vi "HFRR ADV v030 new software.vi"() -> ()   [LabVIEW 2025] (continued)
                n317 = Wait (ms)(milliseconds to wait=u32 1500) -> ()  [unwired: 1 out]
              }
              frame #5 {
                n318 = stacked-sequence {
                  frame #0 {
                    n319 = Wait (ms)(milliseconds to wait=u32 1500) -> ()  [unwired: 1 out]
                  }
                  frame #1 {
                    n320 = local read "Set Temp"() -> (w400:dbl)
                    n321 = Number To Fractional String(number=w400, precision (6)=i16 2) -> (F-format string=w403:string)  [unwired: 2 in]
                    n322 = Concatenate Strings("ST;" ("Command"), w403) -> (w402:string)
                    n323 = local write "Due Write"(w402) -> ()
                  }
                  frame #2 {
                    n324 = Wait (ms)(milliseconds to wait=u32 1500) -> ()  [unwired: 1 out]
                  }
                  frame #3 {
                    n325 = local write "Due Write"("HE;1" ("Command")) -> ()
                  }
                  frame #4 {
                    n326 = Wait (ms)(milliseconds to wait=u32 1500) -> ()  [unwired: 1 out]
                  }
                }
              }
            }
          }
          frame False {
            n327 = stacked-sequence {
              frame #0 {
                n328 = Wait (ms)(milliseconds to wait=u32 1500) -> ()  [unwired: 1 out]
              }
              frame #1 {
                n329 = Concatenate Strings("ST;" ("Command"), "0" ("string")) -> (w410:string)
                n330 = local write "Due Write"(w410) -> ()
              }
              frame #2 {
                n331 = Wait (ms)(milliseconds to wait=u32 1500) -> ()  [unwired: 1 out]
              }
              frame #3 {
                n332 = local write "Due Write"("HE;0" ("Command")) -> ()
              }
              frame #4 {
                n333 = Wait (ms)(milliseconds to wait=u32 1500) -> ()  [unwired: 1 out]
              }
            }
          }
        }
      }
      event "Headen Service Button": Value Change {
        n334 = event-data() -> ()  [unwired: 1 in, 6 out]
        n335 = local read "Headen Service Button"() -> (w415:bool)
        n336 = case shown="True" w415 {
          frame False {
            n337 = property on="Password 3" class="Clust (strict)"("Visible"=FALSE) -> ()  [unwired: 2 in, 2 out]
            n338 = property on="Service Password Log" class="Str"("Visible"=FALSE) -> ()  [unwired: 2 in, 2 out]
          }
          frame True {
            n339 = property on="Password 3" class="Clust (strict)"("Visible"=TRUE) -> ()  [unwired: 2 in, 2 out]
            n340 = property on="Service Password Log" class="Str"("Visible"=TRUE) -> ()  [unwired: 2 in, 2 out]
          }
        }
      }
      event "Password 3.Service Password": Value Change {
        n341 = event-data() -> ()  [unwired: 1 in, 6 out]
        n342 = Unbundle By Name("Password 3") -> ("Service Password"=w422:string)
        n343 = call <vilib>:"Trim Whitespace.vi"("string"=w422) -> ("trimmed string"=w420:string)  [unwired: 1 in]
        n344 = Equal?(x=w420, y="Service@123") -> (x = y?=w421:bool)
        n345 = case shown="False" w421 {
          selector: w421 -> [w425 w427]
          frame False {
            n346 = local write "Service Password enable"(w425) -> ()
            n347 = property on="Service Password Log" class="Str"("Visible"=TRUE) -> ()  [unwired: 2 in, 2 out]
          }
          frame True {
            n348 = property on="Service Password Log" class="Str"("Visible"=FALSE) -> ()  [unwired: 2 in, 2 out]
            "Service Password enable" <- w427
          }
        }
      }
      event "Sign In": Value Change {
        w429 = FALSE ("Visible")
        n349 = event-data() -> ()  [unwired: 1 in, 6 out]
        n350 = property on="About" class="Clust (strict)"("Visible"=w429) -> ()  [unwired: 2 in, 2 out]
        n351 = property on="Password 3" class="Clust (strict)"("Visible"=w429) -> ()  [unwired: 2 in, 2 out]
        n352 = property on="Service Password Log" class="Str"("Visible"=FALSE) -> ()  [unwired: 2 in, 2 out]
      }
      event "Info": Value Change {
        n353 = event-data() -> ()  [unwired: 1 in, 6 out]
        n354 = local read "Info"() -> (w431:bool)
        n355 = case shown="False" w431 {
          frame False {
            n356 = property on="About" class="Clust (strict)"("Visible"=FALSE) -> ()  [unwired: 2 in, 2 out]
          }
          frame True {
            n357 = property on="About" class="Clust (strict)"("Visible"=TRUE) -> ()  [unwired: 2 in, 2 out]
          }
        }
      }
      event "Calibration": Value Change {
        n358 = event-data() -> ()  [unwired: 1 in, 6 out]
        n359 = local read "Calibration"() -> (w435:bool)
        n360 = case shown="False" w435 {
          frame False {
            n361 = property on="Calibration 2" class="TabCtl (strict)"("Visible"=FALSE) -> ()  [unwired: 2 in, 2 out]
            n362 = local write "Cal Password"("" ("Cal Password")) -> ()
          }
          frame True {
            n363 = property on="Calibration 2" class="TabCtl (strict)"("Visible"=TRUE) -> ()  [unwired: 2 in, 2 out]
            n364 = local write "Cal Password"("" ("Cal Password")) -> ()
          }
        }
        n365 = property on="Wrong Password" class="Str"("Visible"=FALSE) -> ()  [unwired: 2 in, 2 out]
      }
      event "Cal Password": Value Change {
        n366 = event-data() -> ()  [unwired: 1 in, 6 out]
        n367 = local read "Cal Password"() -> (w443:string)
        n368 = call <vilib>:"Trim Whitespace.vi"("string"=w443) -> ("trimmed string"=w442:string)  [unwired: 1 in]
        n369 = Equal?(x=w442, y="Cal@321") -> (x = y?=w440:bool)
        n370 = case shown="True" w440 {
          frame False {
            n371 = property on="Wrong Password" class="Str"("Visible"=TRUE) -> ()  [unwired: 2 in, 2 out]
          }
          frame True {
            n372 = property on="Wrong Password" class="Str"("Visible"=FALSE) -> ()  [unwired: 2 in, 2 out]
            n373 = local write "Main Tab"(T2."About" ("Main Tab")) -> ()
            n374 = local write "Cal Password"("" ("Cal Password")) -> ()
            n375 = local write "Main Dashboard Buttons"(T1."About" ("Main Dashboard Buttons")) -> ()
            n376 = property on="Calibration 2" class="TabCtl (strict)"("Visible"=FALSE) -> ()  [unwired: 2 in, 2 out]
            n377 = local write "Calibration"(FALSE ("Calibration")) -> ()
          }
        }
      }
      event "Calibration Selection": Value Change {
        n378 = event-data() -> ()  [unwired: 1 in, 6 out]
        n379 = local read "Calibration Selection"() -> (w452:T8)
        n380 = case shown="\"Stroke Calibration\"" w452 {
          tunnel: [T7."Stroke" ("Main Calibration Tab") T7."Friction" ("Main Calibration Tab") T7."Main" ("Main Calibration Tab") T7."Temperature" ("Main Calibration Tab")] -> w451
          frame "Stroke Calibration" {
          }
          frame "Friction Force Calibration" {
          }
          frame Default {
          }
          frame "Temperature Calibration" {
          }
        }
        n381 = local write "Main Calibration Tab"(w451) -> ()
      }
      event "Back Stroke": Value Change {
        n382 = event-data() -> ()  [unwired: 1 in, 6 out]
        n383 = local write "Main Stroke Tab"(T9."Step 1" ("Main Stroke Tab")) -> ()
        n384 = local write "Main Calibration Tab"(T7."Main" ("Main Calibration Tab")) -> ()
        n385 = local write "Back Stroke"(FALSE ("Back Stroke")) -> ()
      }
      event "Step 2 Back": Value Change {
        n386 = event-data() -> ()  [unwired: 1 in, 6 out]
        n387 = local write "Main Stroke Tab"(T9."Step 1" ("Main Stroke Tab")) -> ()
        n388 = local write "Step 2 Back"(FALSE ("Back Stroke")) -> ()
      }
      event "Step 3 Back": Value Change {
        n389 = event-data() -> ()  [unwired: 1 in, 6 out]
        n390 = local write "Main Stroke Tab"(T9."Step 2" ("Main Stroke Tab")) -> ()
        n391 = local write "Step 3 Back"(FALSE ("Back Stroke")) -> ()
      }
      event "Step 4 Back": Value Change {
        n392 = event-data() -> ()  [unwired: 1 in, 6 out]
        n393 = local write "Main Stroke Tab"(T9."Step 3" ("Main Stroke Tab")) -> ()
        n394 = local write "Step 4 Back"(FALSE ("Back Stroke")) -> ()
      }
      event "Step 5 Back": Value Change {
        n395 = event-data() -> ()  [unwired: 1 in, 6 out]
        n396 = local write "Main Stroke Tab"(T9."Step 4" ("Main Stroke Tab")) -> ()
        n397 = local write "Step 5 Back"(FALSE ("Back Stroke")) -> ()
      }
      event "Step 6 Back": Value Change {
        n398 = event-data() -> ()  [unwired: 1 in, 6 out]
        n399 = local write "Main Stroke Tab"(T9."Step 5" ("Main Stroke Tab")) -> ()
        n400 = local write "Step 6 Back"(FALSE ("Back Stroke")) -> ()
      }
      event "Back Stroke step 7": Value Change {
        n401 = event-data() -> ()  [unwired: 1 in, 6 out]
        n402 = local write "Main Stroke Tab"(T9."Step 6" ("Main Stroke Tab")) -> ()
        n403 = local write "Back Stroke step 7"(FALSE ("Back Stroke")) -> ()
      }
      event "Back Stroke step 8": Value Change {
        n404 = event-data() -> ()  [unwired: 1 in, 6 out]
        n405 = local write "Main Stroke Tab"(T9."Step 7" ("Main Stroke Tab")) -> ()
        n406 = local write "Back Stroke step 8"(FALSE ("Back Stroke")) -> ()
      }
      event "Back Stroke 8": Value Change {
        n407 = event-data() -> ()  [unwired: 1 in, 6 out]
        n408 = local write "MOVE CARRIAGE TO"(0.2 ("MOVE CARRIAGE TO")) -> ()
        n409 = local write "Main Stroke Tab"(T9."Step 1" ("Main Stroke Tab")) -> ()
        n410 = local write "Back Stroke 8"(FALSE ("Back Stroke 8")) -> ()
      }
      event "Continue Stroke": Value Change {
        n411 = event-data() -> ()  [unwired: 1 in, 6 out]
        n412 = local write "Main Stroke Tab"(T9."Step 2" ("Main Stroke Tab")) -> ()
        n413 = local write "Continue Stroke"(FALSE ("Continue Stroke")) -> ()
      }
      event "Continue Stroke step 2": Value Change {
        n414 = event-data() -> ()  [unwired: 1 in, 6 out]
        n415 = local write "Main Stroke Tab"(T9."Step 3" ("Main Stroke Tab")) -> ()
        n416 = local write "Continue Stroke step 2"(FALSE ("Continue Stroke")) -> ()
      }
      event "Continue Stroke step 3": Value Change {
        n417 = event-data() -> ()  [unwired: 1 in, 6 out]
        n418 = local write "Main Stroke Tab"(T9."Step 4" ("Main Stroke Tab")) -> ()
        n419 = local write "Continue Stroke step 3"(FALSE ("Continue Stroke")) -> ()
      }
      event "Continue Stroke step 4": Value Change {
        n420 = event-data() -> ()  [unwired: 1 in, 6 out]
        n421 = local write "Main Stroke Tab"(T9."Step 5" ("Main Stroke Tab")) -> ()
        n422 = local write "Continue Stroke step 4"(FALSE ("Continue Stroke")) -> ()
      }
      event "Continue Stroke step 5": Value Change {
        n423 = event-data() -> ()  [unwired: 1 in, 6 out]
        n424 = local write "Main Stroke Tab"(T9."Step 6" ("Main Stroke Tab")) -> ()
        n425 = local write "Continue Stroke step 5"(FALSE ("Continue Stroke")) -> ()
      }
      event "Continue Stroke step 6": Value Change {
        n426 = event-data() -> ()  [unwired: 1 in, 6 out]
        n427 = local write "Main Stroke Tab"(T9."Step 7" ("Main Stroke Tab")) -> ()
        n428 = local write "Continue Stroke step 6"(FALSE ("Continue Stroke")) -> ()
      }
      event "Continue Stroke step 7": Value Change {
        w491 = FALSE ("0.2mm")
        n429 = event-data() -> ()  [unwired: 1 in, 6 out]
        n430 = local write "0.4 mm"(w491) -> ()
        n431 = local write "0.6 mm"(w491) -> ()
        n432 = local write "1.0 mm"(w491) -> ()
        n433 = local write "1.2 mm"(w491) -> ()
        n434 = local write "0.2 2"(w491) -> ()
        n435 = local write "0.4 2"(w491) -> ()
        n436 = local write "0.6 2"(w491) -> ()
        n437 = local write "0.8 2"(w491) -> ()
        n438 = local write "1.0 2"(w491) -> ()
        n439 = local write "1.2"(w491) -> ()
        n440 = local write "0.2mm"(w491) -> ()
        n441 = local write "0.8mm"(w491) -> ()
        n442 = local write "Main Stroke Tab"(T9."Step 8" ("Main Stroke Tab")) -> ()
        n443 = local write "Continue Stroke step 7"(FALSE ("Continue Stroke")) -> ()
        n444 = local write "Stroke Test Complete"(T10."Test Progress" ("Stroke Test Complete")) -> ()
        "Position Measurment Temp" <- 0.0 ("Position Measurment Temp")
        "Calibration Tare" <- TRUE ("Calibration Tare")
        "MOVE CARRIAGE TO" <- 0.2 ("MOVE CARRIAGE TO")
      }
      event "Continue Stroke step 8": Value Change {
        n445 = event-data() -> ()  [unwired: 1 in, 6 out]
        n446 = local read "LVDT STROKE  Calibration"() -> (w496:dbl)
        n447 = local read "Position Measurment Temp"() -> (w497:dbl)
        n448 = case shown="7" w497 {
          selector: w497 -> [w502 w507 w512 w517 w522 w526 w529 w530]
          tunnel: w496 -> [w498 w503 w508 w513 w518 w523 _ _]
          frame 0, Default {
            w500 = TRUE ("0.2mm")
            n449 = Increment(x=w502) -> (x+1=w501:i32)
            n450 = local write "Position Measurment Temp"(w501) -> ()
            n451 = local write "0.2mm"(w500) -> ()
            n452 = local write "0.2 2"(w500) -> ()
            n453 = local write "MOVE CARRIAGE TO"(0.4 ("MOVE CARRIAGE TO")) -> ()
            "Calibration 0.2" <- w498
          }
          frame 1 {
            w505 = TRUE ("0.4 mm")
            n454 = Increment(x=w507) -> (x+1=w506:i32)
            n455 = local write "Calibration 0.4"(w503) -> ()
            n456 = local write "Position Measurment Temp"(w506) -> ()
            n457 = local write "0.4 mm"(w505) -> ()
            n458 = local write "MOVE CARRIAGE TO"(0.6 ("MOVE CARRIAGE TO")) -> ()
            n459 = local write "0.4 2"(w505) -> ()
          }
          frame 2 {
            w510 = TRUE ("0.6 mm")
            n460 = Increment(x=w512) -> (x+1=w511:i32)
            n461 = local write "Calibration 0.6"(w508) -> ()
            n462 = local write "Position Measurment Temp"(w511) -> ()
            n463 = local write "0.6 2"(w510) -> ()
            n464 = local write "0.6 mm"(w510) -> ()
            n465 = local write "MOVE CARRIAGE TO"(0.8 ("MOVE CARRIAGE TO")) -> ()
          }
          frame 3 {
            w514 = TRUE ("0.6 mm")
            n466 = Increment(x=w517) -> (x+1=w516:i32)
            n467 = local write "Position Measurment Temp"(w516) -> ()
            n468 = local write "MOVE CARRIAGE TO"(1.0 ("MOVE CARRIAGE TO")) -> ()
            n469 = local write "0.8mm"(w514) -> ()
            n470 = local write "0.8 2"(w514) -> ()
            "Calibration 0.8" <- w513
          }
          frame 4 {
            w519 = TRUE ("0.6 mm")
            n471 = Increment(x=w522) -> (x+1=w521:i32)
            n472 = local write "Position Measurment Temp"(w521) -> ()
            n473 = local write "MOVE CARRIAGE TO"(1.2 ("MOVE CARRIAGE TO")) -> ()
            n474 = local write "1.0 mm"(w519) -> ()
            n475 = local write "1.0 2"(w519) -> ()
            "Calibration 1.0" <- w518
          }
          frame 5 {
            w524 = TRUE ("0.6 mm")
            n476 = Increment(x=w526) -> (x+1=w525:i32)
            n477 = local write "Position Measurment Temp"(w525) -> ()
            n478 = local write "1.2 mm"(w524) -> ()
            n479 = local write "1.2"(w524) -> ()
            "Calibration 1.2" <- w523
          }
          frame 6 {
            n480 = Increment(x=w529) -> (x+1=w528:i32)
            n481 = local write "Position Measurment Temp"(w528) -> ()
            n482 = local write "Stroke Test Complete"(T10."Stroke Points Completed" ("Stroke Test Complete")) -> ()
          }
          frame 7 {
            n483 = stacked-sequence {
              tunnel: w530 -> [w531 _ _]
              frame #0 {
                n484 = Increment(x=w531) -> (x+1=w532:i32)
                n485 = local write "Main Stroke Tab"(T9."Step 9" ("Main Stroke Tab")) -> ()
                n486 = local write "Position Measurment Temp"(w532) -> ()
                n487 = Insert Into Array(array=dbl[] [], new element #1=0.2 ("new element/subarray"), new element #2=0.4 ("new element/subarray"), new element #3=0.6 ("new element/subarray"), new element #4=0.8 ("new element/subarray"), new element #5=1.0 ("new element/subarray"), new element #6=1.2 ("new element/subarray")) -> (→"1D stroke":dbl[])  [unwired: 1 in]
                n488 = local read "Calibration 0.2"() -> (w539:dbl)
                n489 = local read "Calibration 0.4"() -> (w538:dbl)
                n490 = local read "Calibration 0.6"() -> (w537:dbl)
                n491 = local read "Calibration 0.8"() -> (w536:dbl)
                n492 = local read "Calibration 1.0"() -> (w535:dbl)
                n493 = local read "Calibration 1.2"() -> (w534:dbl)
                n494 = Insert Into Array(array=dbl[] [], new element #1=w539, new element #2=w538, new element #3=w537, new element #4=w536, new element #5=w535, new element #6=w534) -> (→"Calibrated Voltage Value":dbl[])  [unwired: 1 in]
              }
              frame #1 {
                n495 = local read "calibration values"() -> (w562:dbl[])
                n496 = local read "Calibrated Voltage Value"() -> (w564:dbl[])
                n497 = Index Array(array=w562, index #1=1 ("index"), index #2=3 ("index"), index #3=5 ("index"), index #4=7 ("index"), index #5=9 ("index"), index #6=11 ("index")) -> (element #1=w555:dbl, element #2=w554:dbl, element #3=w553:dbl, element #4=w552:dbl, element #5=w551:dbl, element #6=w550:dbl)
                n498 = local read "1D stroke"() -> (w565:dbl[])
                n499 = for {
                  tunnel: [w574] -> w563 mode=indexing
                  tunnel: w565 -> [w573] mode=indexing
                  tunnel: w564 -> [w572] mode=indexing
                  tunnel: w555 -> [w571]
                  tunnel: w554 -> [w570]
                  tunnel: w553 -> [w569]
                  tunnel: w552 -> [w568]
                  tunnel: w551 -> [w567]
                  tunnel: w550 -> [w566]
                  n500 = formula code="if (stroke == 0.2)\n{\n    if ((voltage >= REF_02 - 0.2) && (voltage <= REF_02 + 0.2))\n        status = 1;\n    else\n        status = 0;\n}\nelse if (stroke == 0.4)\n{\n    if ((voltage >= REF_04 - 0.2) && (voltage <= REF_04 + 0.2))\n        status = 1;\n    else\n        status = 0;\n}\nelse if (stroke == 0.6)\n{\n    if ((voltage >= REF_06 - 0.2) && (voltage <= REF_06 + 0.2))\n        status = 1;\n    else\n        status = 0;\n}\nelse if (stroke == 0.8)\n{\n    if ((voltage >= REF_08 - 0.2) && (voltage <= REF_08 + 0.2))\n        status = 1;\n    else\n        status = 0;\n}\nelse if (stroke == 1.0)\n{\n    if ((voltage >= REF_10 - 0.2) && (voltage <= REF_10 + 0.2))\n        status = 1;\n    else\n        status = 0;\n}\nelse if (stroke == 1.2)\n{\n    if ((voltage >= REF_12 - 0.2) && (voltage <= REF_12 + 0.2))\n        status = 1;\n    else\n        status = 0;\n}\nelse\n{\n    status = 0;\n}"("stroke"=w573, "voltage"=w572, "REF_02"=w571, "REF_04"=w570, "REF_06"=w569, "REF_08"=w568, "REF_10"=w567, "REF_12"=w566) -> ("status"=w574:dbl)
                }
                "Status" <- w563
              }
              frame #2 {
                w581 = 1.0
                n501 = local read "Status"() -> (w588:dbl[])
                n502 = Index Array(array=w588) -> (element #1=w587:dbl, element #2=w586:dbl, element #3=w585:dbl, element #4=w584:dbl, element #5=w583:dbl, element #6=w582:dbl)  [unwired: 6 in]
                n503 = Equal?(x=w586, y=w581) -> (x = y?=w579:bool)
                n504 = Equal?(x=w585, y=w581) -> (x = y?=w578:bool)
                n505 = Equal?(x=w584, y=w581) -> (x = y?=w577:bool)
                n506 = Equal?(x=w583, y=w581) -> (x = y?=w576:bool)
                n507 = Equal?(x=w582, y=w581) -> (x = y?=w575:bool)
                n508 = Equal?(x=w587, y=w581) -> (x = y?=w580:bool)
                n509 = case shown="True" w580 {
                  selector: w580 -> [w599 w600]
                  frame True {
                    n510 = local write "Point 1 - 0.2 mm"(w599) -> ()
                    n511 = property on="Point 1 - 0.2 mm" class="Bool"("Caption.Visible"=w599) -> ()  [unwired: 2 in, 2 out]
                  }
                  frame False {
                    n512 = local write "Point 1 - 0.2 mm"(w600) -> ()
                    n513 = property on="Point 1 - 0.2 mm" class="Bool"("Caption.Visible"=w600) -> ()  [unwired: 2 in, 2 out]
                  }
                }
                n514 = case shown="True" w579 {
                  selector: w579 -> [w597 w598]
                  frame True {
                    n515 = local write "Point 2 - 0.4 mm"(w597) -> ()
                    n516 = property on="Point 2 - 0.4 mm" class="Bool"("Caption.Visible"=w597) -> ()  [unwired: 2 in, 2 out]
                  }
                  frame False {
                    n517 = local write "Point 2 - 0.4 mm"(w598) -> ()
                    n518 = property on="Point 2 - 0.4 mm" class="Bool"("Caption.Visible"=w598) -> ()  [unwired: 2 in, 2 out]
                  }
                }
                n519 = case shown="True" w576 {
                  selector: w576 -> [w591 w592]
                  frame True {
                    n520 = local write "Point 5 - 1.0 mm"(w591) -> ()
                    n521 = property on="Point 5 - 1.0 mm" class="Bool"("Caption.Visible"=w591) -> ()  [unwired: 2 in, 2 out]
                  }
                  frame False {
                    n522 = local write "Point 5 - 1.0 mm"(w592) -> ()
                    n523 = property on="Point 5 - 1.0 mm" class="Bool"("Caption.Visible"=w592) -> ()  [unwired: 2 in, 2 out]
                  }
                }
                n524 = case shown="True" w578 {
                  selector: w578 -> [w595 w596]
                  frame True {
                    n525 = local write "Point 3 - 0.6 mm"(w595) -> ()
                    n526 = property on="Point 3 - 0.6 mm" class="Bool"("Caption.Visible"=w595) -> ()  [unwired: 2 in, 2 out]
                  }
                  frame False {
                    n527 = local write "Point 3 - 0.6 mm"(w596) -> ()
                    n528 = property on="Point 3 - 0.6 mm" class="Bool"("Caption.Visible"=w596) -> ()  [unwired: 2 in, 2 out]
                  }
                }
                n529 = case shown="True" w577 {
                  selector: w577 -> [w593 w594]
                  frame True {
                    n530 = local write "Point 4 - 0.8 mm"(w593) -> ()
                    n531 = property on="Point 4 - 0.8 mm" class="Bool"("Caption.Visible"=w593) -> ()  [unwired: 2 in, 2 out]
                  }
                  frame False {
                    n532 = local write "Point 4 - 0.8 mm"(w594) -> ()
                    n533 = property on="Point 4 - 0.8 mm" class="Bool"("Caption.Visible"=w594) -> ()  [unwired: 2 in, 2 out]
                  }
                }
                n534 = case shown="True" w575 {
                  selector: w575 -> [w589 w590]
                  frame True {
                    n535 = local write "Point 6 - 1.2 mm"(w589) -> ()
                    n536 = property on="Point 6 - 1.2 mm" class="Bool"("Caption.Visible"=w589) -> ()  [unwired: 2 in, 2 out]
                  }
                  frame False {
                    n537 = local write "Point 6 - 1.2 mm"(w590) -> ()
                    n538 = property on="Point 6 - 1.2 mm" class="Bool"("Caption.Visible"=w590) -> ()  [unwired: 2 in, 2 out]
                  }
                }
              }
            }
          }
        }
      }
      event "TEMPERATURE STEP Back 1", "TEMPERATURE STEP Back air Temp": Value Change {
        n539 = event-data() -> ()  [unwired: 1 in, 6 out]
        n540 = stacked-sequence {
          frame #0 {
            n541 = local write "Main Calibration Tab"(T7."Main" ("Main Calibration Tab")) -> ()
          }
          frame #1 {
            n542 = Wait (ms)(milliseconds to wait=u32 1000) -> ()  [unwired: 1 out]
          }
          frame #2 {
            n543 = local write "Due Write"("CAL;END" ("Command")) -> ()
          }
          frame #3 {
            n544 = Wait (ms)(milliseconds to wait=u32 2000) -> ()  [unwired: 1 out]
          }
          frame #4 {
            n545 = local write "Due Write"("CAL;END" ("Command")) -> ()
          }
        }
      }
      event "Temperature Continue Step 1": Value Change {
        n546 = event-data() -> ()  [unwired: 1 in, 6 out]
        n547 = stacked-sequence {
          frame #0 {
            n548 = Wait (ms)(milliseconds to wait=u32 1500) -> ()  [unwired: 1 out]
          }
          frame #1 {
            n549 = local write "Due Write"("CAL;START" ("Command")) -> ()
          }
          frame #2 {
            n550 = Wait (ms)(milliseconds to wait=u32 1500) -> ()  [unwired: 1 out]
          }
          frame #3 {
            n551 = local write "Due Write"("CAL;START" ("Command")) -> ()
          }
          frame #4 {
            n552 = Wait (ms)(milliseconds to wait=u32 2000) -> ()  [unwired: 1 out]
          }
          frame #5 {
          }
          frame #6 {
            n553 = Wait (ms)(milliseconds to wait=u32 2000) -> ()  [unwired: 1 out]
          }
          frame #7 {
            # "CAL;A1;<true_T>"
            n554 = local write "Due Write"("CAL;A1;0" ("Command")) -> ()
          }
          frame #8 {
            n555 = local write "Tab Control 4"(T12."Step 2" ("Tab Control 4")) -> ()
          }
        }
      }
      event "Temperature Continue Step air Step 1": Value Change {
        n556 = event-data() -> ()  [unwired: 1 in, 6 out]
        n557 = stacked-sequence {
          frame #0 {
            n558 = Wait (ms)(milliseconds to wait=u32 1500) -> ()  [unwired: 1 out]
          }
          frame #1 {
            n559 = local write "Due Write"("CAL;START" ("Command")) -> ()
          }
          frame #2 {
            n560 = Wait (ms)(milliseconds to wait=u32 1500) -> ()  [unwired: 1 out]
          }
          frame #3 {
            n561 = local write "Due Write"("CAL;START" ("Command")) -> ()
          }
          frame #4 {
            n562 = Wait (ms)(milliseconds to wait=u32 2000) -> ()  [unwired: 1 out]
          }
          frame #5 {
          }
          frame #6 {
            n563 = Wait (ms)(milliseconds to wait=u32 2000) -> ()  [unwired: 1 out]
          }
          frame #7 {
            # "CAL;A1;<true_T>"
            n564 = local write "Due Write"("CAL;A1;0" ("Command")) -> ()
          }
          frame #8 {
            n565 = local write "Tab Control 4"(T12."Air Step 2" ("Tab Control 4")) -> ()
          }
        }
      }
      event "Temperature Selection": Value Change {
        n566 = event-data() -> ()  [unwired: 1 in, 6 out]
        n567 = local read "Temperature Selection"() -> (w622:T13)
        n568 = case shown="\"Default\", Default" w622 {
          frame "Air Temperature" {
            n569 = local write "Tab Control 4"(T12."Air Step 1" ("Tab Control 4")) -> ()
          }
          frame "Sample Temperature" {
            n570 = local write "Tab Control 4"(T12."Step 1" ("Tab Control 4")) -> ()
          }
          frame "Default", Default {
          }
        }
      }
      event "Temperature Continue Step 2": Value Change {
        n571 = event-data() -> ()  [unwired: 1 in, 6 out]
        n572 = stacked-sequence {
          frame #0 {
            n573 = stacked-sequence {
              frame #0 {
                n574 = Wait (ms)(milliseconds to wait=u32 1500) -> ()  [unwired: 1 out]
              }
              frame #1 {
                # "CAL;A1;<true_T>"
                n575 = local write "Due Write"("CAL;A1;0" ("Command")) -> ()
              }
              frame #2 {
                n576 = Wait (ms)(milliseconds to wait=u32 1500) -> ()  [unwired: 1 out]
              }
              frame #3 {
                # "CAL;A1;<true_T>"
                n577 = local write "Due Write"("CAL;A1;0" ("Command")) -> ()
              }
              frame #4 {
              }
            }
          }
          frame #1 {
            n578 = local write "Tab Control 4"(T12."Step 3" ("Tab Control 4")) -> ()
          }
        }
      }
      event "Temperature Continue Step 5": Value Change {
        n579 = event-data() -> ()  [unwired: 1 in, 6 out]
        n580 = stacked-sequence {
          frame #0 {
            n581 = stacked-sequence {
              frame #0 {
                n582 = Wait (ms)(milliseconds to wait=u32 1500) -> ()  [unwired: 1 out]
              }
              frame #1 {
                # "CAL;A1;<true_T>"
                n583 = local write "Due Write"("CAL;A1;0" ("Command")) -> ()
              }
              frame #2 {
                n584 = Wait (ms)(milliseconds to wait=u32 1500) -> ()  [unwired: 1 out]
              }
              frame #3 {
                # "CAL;A1;<true_T>"
                n585 = local write "Due Write"("CAL;A1;0" ("Command")) -> ()
              }
              frame #4 {
              }
            }
          }
          frame #1 {
            n586 = local write "Tab Control 4"(T12."Air Step 3" ("Tab Control 4")) -> ()
          }
        }
      }
      event "Temperature Continue Step 3": Value Change {
        n587 = event-data() -> ()  [unwired: 1 in, 6 out]
        n588 = stacked-sequence {
          frame #0 {
            n589 = stacked-sequence {
              frame #0 {
                n590 = Wait (ms)(milliseconds to wait=u32 1500) -> ()  [unwired: 1 out]
              }
              frame #1 {
              }
              frame #2 {
              }
              frame #3 {
                # "CAL;A1;<true_T>"
                n591 = local write "Due Write"("CAL;A1;60" ("Command")) -> ()
              }
              frame #4 {
                n592 = Wait (ms)(milliseconds to wait=u32 2000) -> ()  [unwired: 1 out]
              }
              frame #5 {
                # "CAL;A1;<true_T>"
                n593 = local write "Due Write"("CAL;A1;60" ("Command")) -> ()
              }
            }
          }
          frame #1 {
            n594 = Wait (ms)(milliseconds to wait=u32 1000) -> ()  [unwired: 1 out]
          }
          frame #2 {
            n595 = local write "Due Write"("CAL;SAVE" ("Command")) -> ()
          }
          frame #3 {
            n596 = Wait (ms)(milliseconds to wait=u32 1000) -> ()  [unwired: 1 out]
          }
          frame #4 {
            n597 = local write "Due Write"("CAL;SAVE" ("Command")) -> ()
          }
          frame #5 {
            n598 = Wait (ms)(milliseconds to wait=u32 1000) -> ()  [unwired: 1 out]
          }
          frame #6 {
            # "CAL;END"
            n599 = local write "Due Write"("CAL;END" ("Command")) -> ()
          }
          frame #7 {
            n600 = Wait (ms)(milliseconds to wait=u32 1000) -> ()  [unwired: 1 out]
          }
          frame #8 {
            # "CAL;END"
            n601 = local write "Due Write"("CAL;END" ("Command")) -> ()
          }
          frame #9 {
            n602 = local write "Main Calibration Tab"(T7."Temperature" ("Main Calibration Tab")) -> ()
            n603 = local write "Tab Control 4"(T12."Main" ("Tab Control 4")) -> ()
          }
        }
      }
      event "Temperature Continue Step 6": Value Change {
        n604 = event-data() -> ()  [unwired: 1 in, 6 out]
        n605 = stacked-sequence {
          frame #0 {
            n606 = stacked-sequence {
              frame #0 {
                n607 = Wait (ms)(milliseconds to wait=u32 1500) -> ()  [unwired: 1 out]
              }
              frame #1 {
              }
              frame #2 {
              }
              frame #3 {
                # "CAL;A1;<true_T>"
                n608 = local write "Due Write"("CAL;A1;60" ("Command")) -> ()
              }
              frame #4 {
                n609 = Wait (ms)(milliseconds to wait=u32 2000) -> ()  [unwired: 1 out]
              }
              frame #5 {
                # "CAL;A1;<true_T>"
                n610 = local write "Due Write"("CAL;A1;60" ("Command")) -> ()
              }
            }
          }
          frame #1 {
            n611 = Wait (ms)(milliseconds to wait=u32 1000) -> ()  [unwired: 1 out]
          }
          frame #2 {
            n612 = local write "Due Write"("CAL;SAVE" ("Command")) -> ()
          }
          frame #3 {
            n613 = Wait (ms)(milliseconds to wait=u32 1000) -> ()  [unwired: 1 out]
          }
          frame #4 {
            n614 = local write "Due Write"("CAL;SAVE" ("Command")) -> ()
          }
          frame #5 {
            n615 = Wait (ms)(milliseconds to wait=u32 1000) -> ()  [unwired: 1 out]
          }
          frame #6 {
            # "CAL;END"
            n616 = local write "Due Write"("CAL;END" ("Command")) -> ()
          }
          frame #7 {
            n617 = Wait (ms)(milliseconds to wait=u32 1000) -> ()  [unwired: 1 out]
          }
          frame #8 {
            # "CAL;END"
            n618 = local write "Due Write"("CAL;END" ("Command")) -> ()
          }
          frame #9 {
            n619 = local write "Main Calibration Tab"(T7."Temperature" ("Main Calibration Tab")) -> ()
            n620 = local write "Tab Control 4"(T12."Main" ("Tab Control 4")) -> ()
          }
        }
      }
      event "Back Stroke step main temperature": Value Change {
        n621 = event-data() -> ()  [unwired: 1 in, 6 out]
        n622 = stacked-sequence {
          frame #0 {
            n623 = Wait (ms)(milliseconds to wait=u32 1000) -> ()  [unwired: 1 out]
          }
          frame #1 {
            # "CAL;END"
            n624 = local write "Due Write"("CAL;END" ("Command")) -> ()
          }
          frame #2 {
            n625 = Wait (ms)(milliseconds to wait=u32 1000) -> ()  [unwired: 1 out]
          }
          frame #3 {
            # "CAL;END"
            n626 = local write "Due Write"("CAL;END" ("Command")) -> ()
          }
          frame #4 {
            n627 = local write "Main Calibration Tab"(T7."Main" ("Main Calibration Tab")) -> ()
            n628 = local write "Tab Control 4"(T12."Main" ("Tab Control 4")) -> ()
          }
        }
      }
      event "TEMPERATURE STEP  Back 4", "TEMPERATURE STEP 1 Back 3", "TEMPERATURE STEP  Back 3", "TEMPERATURE STEP 1 Back 2": Value Change {
        # "Back Stroke step main temperature"
        n629 = event-data() -> ()  [unwired: 1 in, 6 out]
        n630 = stacked-sequence {
          frame #0 {
            n631 = Wait (ms)(milliseconds to wait=u32 1000) -> ()  [unwired: 1 out]
          }
          frame #1 {
            # "CAL;END"
            n632 = local write "Due Write"("CAL;END" ("Command")) -> ()
          }
          frame #2 {
            n633 = Wait (ms)(milliseconds to wait=u32 1000) -> ()  [unwired: 1 out]
          }
          frame #3 {
            # "CAL;END"
            n634 = local write "Due Write"("CAL;END" ("Command")) -> ()
          }
          frame #4 {
            # "TEMPERATURE STEP  Back 4"
            n635 = local write "Main Calibration Tab"(T7."Temperature" ("Main Calibration Tab")) -> ()
            n636 = local write "Tab Control 4"(T12."Main" ("Tab Control 4")) -> ()
          }
        }
      }
      event "FF BACK", "FF BACK 2", "FF BACK 3", "FF BACK 4", "FF BACK 5", "FF BACK 6": Value Change {
        n637 = event-data() -> ()  [unwired: 1 in, 6 out]
        n638 = stacked-sequence {
          frame #0 {
            n639 = Wait (ms)(milliseconds to wait=u32 1500) -> ()  [unwired: 1 out]
          }
          frame #1 {
            n640 = local write "Due Write"("VC;0") -> ()
          }
          frame #2 {
            n641 = Wait (ms)(milliseconds to wait=u32 1500) -> ()  [unwired: 1 out]
          }
          frame #3 {
            n642 = local write "Due Write"("VC;0") -> ()
          }
          frame #4 {
            w679 = FALSE
            n643 = local write "FF BACK 2"(w679) -> ()
            n644 = local write "FF BACK 3"(w679) -> ()
            n645 = local write "FF BACK 4"(w679) -> ()
            n646 = local write "FF BACK 5"(w679) -> ()
            n647 = local write "FF BACK 6"(w679) -> ()
            n648 = local write "FF BACK"(w679) -> ()
          }
          frame #5 {
            n649 = local write "Friction Force Tab"(T11."Page 1" ("Friction Force Tab")) -> ()
            n650 = local write "Main Calibration Tab"(T7."Main" ("Main Calibration Tab")) -> ()
          }
        }
      }
      event "FF CONTINUE": Value Change {
        n651 = event-data() -> ()  [unwired: 1 in, 6 out]
        n652 = local write "FF CONTINUE"(FALSE ("FF CONTINUE")) -> ()
        n653 = local write "Friction Force Tab"(T11."Page 2" ("Friction Force Tab")) -> ()
      }
      event "FF CONTINUE 2": Value Change {
        n654 = event-data() -> ()  [unwired: 1 in, 6 out]
        n655 = local write "FF CONTINUE 2"(FALSE ("FF CONTINUE")) -> ()
        n656 = local write "Friction Force Tab"(T11."Page 3" ("Friction Force Tab")) -> ()
      }
      event "FF CONTINUE 3": Value Change {
        n657 = event-data() -> ()  [unwired: 1 in, 6 out]
        n658 = local write "FF CONTINUE 3"(FALSE ("FF CONTINUE")) -> ()
        n659 = local write "Friction Force Tab"(T11."Page 4" ("Friction Force Tab")) -> ()
      }
      event "FF CONTINUE 4": Value Change {
        n660 = event-data() -> ()  [unwired: 1 in, 6 out]
        n661 = local write "FF CONTINUE 4"(FALSE ("FF CONTINUE")) -> ()
        n662 = local write "Friction Force Tab"(T11."Page 5" ("Friction Force Tab")) -> ()
      }
      event "FF CONTINUE 5": Value Change {
        n663 = event-data() -> ()  [unwired: 1 in, 6 out]
        n664 = local write "FF CONTINUE 5"(FALSE ("FF CONTINUE")) -> ()
        n665 = local write "Friction Force Tab"(T11."Page 6" ("Friction Force Tab")) -> ()
      }
      event "Quit": Value Change {
        n666 = event-data() -> ()  [unwired: 1 in, 6 out]
      }
    }
    n667 = Wait (ms)(milliseconds to wait=u32 100) -> ()  [unwired: 1 out]
  }
  n668 = while {
    stop <- w712 stop-if-true
    n669 = local read "Ambient Temperature"() -> (w710:dbl)
    n670 = local read "Sample Temperature"() -> (w709:dbl)
    n671 = Wait (ms)(milliseconds to wait=u32 200) -> ()  [unwired: 1 out]
    n672 = local write "Temperature — Live (Set A: 0 °C)"(w710) -> ()
    n673 = local write "Temperature — Live (Set A: 60 °C)"(w710) -> ()
    n674 = local write "Sensor value"(w710) -> ()
    n675 = local write "Sensor value"(w710) -> ()
    n676 = local write "Sensor value"(w709) -> ()
    n677 = local write "Sensor value"(w709) -> ()
    n678 = local write "Temperature — Live (Set A: 60 °C)"(w709) -> ()
    n679 = local write "Temperature — Live (Set A: 0 °C)"(w709) -> ()
    n680 = case shown="True" "Save Button" {
      selector: "Save Button" -> [_ w727]
      frame False {
      }
      frame True {
        n681 = Not(x=w727) -> (.not. x?=w726:bool)
        n682 = local read "milliseconds to wait"() -> (w759:u32)
        n683 = local read "max_step_change"() -> (w764:dbl)
        n684 = local read "max_amplitude"() -> (w765:dbl)
        n685 = local read "min_amplitude"() -> (w766:dbl)
        n686 = local read "PIEZO_CAL_FACTOR"() -> (w770:dbl)
        n687 = local write "Save Button"(w726) -> ()
        n688 = local read "startup_cmd"() -> (w767:dbl)
        n689 = local read "NORMAL_FORCE"() -> (w771:dbl)
        n690 = local read "ADC_Resolution"() -> (w769:dbl)
        n691 = local read "calibration values"() -> (w774:dbl[])
        n692 = local read "kp"() -> (w761:dbl)
        n693 = local read "kd"() -> (w763:dbl)
        n694 = local read "dt"() -> (w760:dbl)
        n695 = local read "ki"() -> (w762:dbl)
        n696 = local read "STROKE FILTER"() -> (w772:i32)
        n697 = local read "Add up Stroke"() -> (w773:dbl)
        n698 = local read "VREF"() -> (w768:dbl)
        n699 = Insert Into Array(array=dbl[] [], new element #1=w759, new element #2=w760, new element #3=w761, new element #4=w762, new element #5=w763, new element #6=w764, new element #7=w765, new element #8=w766, new element #9=w767) -> (w775:dbl[])  [unwired: 1 in]
        n700 = Insert Into Array(array=dbl[] [], new element #1=w768, new element #2=w769, new element #3=w770, new element #4=w771) -> (w776:dbl[])  [unwired: 1 in]
        n701 = Array To Spreadsheet String(delimiter (Tab)=";", array=w774, 3:"" ("format string")) -> (spreadsheet string=w778:string)
        n702 = Insert Into Array(array=dbl[] [], new element #1=w772, new element #2=w773) -> (w777:dbl[])  [unwired: 1 in]
        n703 = call "Write Config.vi"("Stroke Calibration"=w778, "STROKE PARAMETERS"=w777, "ADC PARAMETERS"=w776, "PID  PARAMETERS"=w775) -> ("error out"=w757:errorcluster)  [unwired: 7 in]
        n704 = call "Stall Data Flow.vim"("value in"=w757, "milliseconds to wait"=u32 2000) -> ("value out"=w758:errorcluster)  [unwired: 1 out]
        n705 = call "Read Config.vi"("error in (no error)"=w758) -> ("STROKE PARAMETERS"=w755:dbl[], "ADC PARAMETERS"=w754:dbl[], "PID  PARAMETERS"=w753:dbl[], "Stroke Calibration"=w756:string)  [unwired: 6 in, 1 out]
        n706 = Index Array(array=w753) -> (element #1=w751:dbl, element #2=w750:dbl, element #3=w749:dbl, element #4=w748:dbl, element #5=w747:dbl, element #6=w746:dbl, element #7=w745:dbl, element #8=w744:dbl, element #9=w743:dbl)  [unwired: 9 in]
        n707 = Index Array(array=w754) -> (element #1=w742:dbl, element #2=w741:dbl, element #3=w740:dbl, element #4=w739:dbl)  [unwired: 4 in]
        n708 = Index Array(array=w755) -> (element #1=w738:dbl, element #2=w737:dbl)  [unwired: 2 in]
        n709 = Spreadsheet String To Array(delimiter (Tab)=";", format string="", spreadsheet string=w756, array type (2D Dbl)=dbl[] []) -> (array=w752:dbl[])
        n710 = local write "VREF"(w742) -> ()
        n711 = local write "ADC_Resolution"(w741) -> ()
        n712 = local write "PIEZO_CAL_FACTOR"(w740) -> ()
        n713 = local write "NORMAL_FORCE"(w739) -> ()
        n714 = local write "STROKE FILTER"(w738) -> ()
        n715 = local write "Add up Stroke"(w737) -> ()
        n716 = local write "calibration values"(w752) -> ()
        n717 = local write "milliseconds to wait"(w751) -> ()
        n718 = local write "dt"(w750) -> ()
        n719 = local write "kp"(w749) -> ()
        n720 = local write "ki"(w748) -> ()
        n721 = local write "kd"(w747) -> ()
        n722 = local write "max_step_change"(w746) -> ()
        n723 = local write "max_amplitude"(w745) -> ()
        n724 = local write "min_amplitude"(w744) -> ()
        n725 = local write "startup_cmd"(w743) -> ()
      }
    }
    n726 = local read "USER ID"() -> (w707:string)
    n727 = local write "tested by 2"(w707) -> ()
    n728 = local read "run test Calibration"() -> (w695:bool)
    n729 = local read "START TEMP"() -> (w694:bool)
    n730 = local read "Point 1 - 0.2 mm"() -> (w706:bool)
    n731 = local read "Point 2 - 0.4 mm"() -> (w705:bool)
    n732 = local read "Point 3 - 0.6 mm"() -> (w704:bool)
    n733 = local read "Point 4 - 0.8 mm"() -> (w703:bool)
    n734 = local read "Point 5 - 1.0 mm"() -> (w702:bool)
    n735 = local read "Point 6 - 1.2 mm"() -> (w701:bool)
    n736 = And(x=w694, y=w695) -> (x .and. y?=w693:bool)
    n737 = And(x=w706, y=w705) -> (x .and. y?=w700:bool)
    n738 = And(x=w704, y=w703) -> (x .and. y?=w699:bool)
    n739 = And(x=w702, y=w701) -> (x .and. y?=w697:bool)
    n740 = case shown="True" w693 {
      frame False {
        w713 = TRUE ("PAUSE")
        n741 = call "ELAPSED TIMER VI - Calibration.vi"("RESET"=w713, "PAUSE"=w713) -> ()  [unwired: 7 in, 3 out]
      }
      frame True {
        w716 = FALSE ("PAUSE")
        n742 = call "ELAPSED TIMER VI - Calibration.vi"("TARGET"=60.0, "RESET"=w716, "PAUSE"=w716) -> ("ELAPSED INDICATION"=w714:bool)  [unwired: 6 in, 2 out]
        n743 = case shown="True" w714 {
          frame False {
          }
          frame True {
            n744 = stacked-sequence {
              frame #0 {
                n745 = local write "START TEMP"(FALSE ("START TEMP")) -> ()
              }
              frame #1 {
                n746 = Wait (ms)(milliseconds to wait=u32 1500) -> ()  [unwired: 1 out]
              }
              frame #2 {
                n747 = local write "Due Write"("VC;0") -> ()
              }
              frame #3 {
                n748 = Wait (ms)(milliseconds to wait=u32 1500) -> ()  [unwired: 1 out]
              }
              frame #4 {
                n749 = local write "Due Write"("VC;0") -> ()
              }
            }
          }
        }
      }
    }
    n750 = And(x=w700, y=w699) -> (x .and. y?=w698:bool)
    n751 = And(x=w698, y=w697) -> (x .and. y?=w696:bool)
    n752 = case shown="False" w696 {
      frame False {
        n753 = property on="Accept & Save" class="Bool (strict)"("DisabledEnum"=T19."Disabled" ("Disabled")) -> ()  [unwired: 2 in, 2 out]
        n754 = property on="Tab Control 5" class="TabCtl (strict)"("Value"=enum32{"OK", "NG"}."NG" ("Tab Control 5")) -> ()  [unwired: 2 in, 2 out]
      }
      frame True {
        n755 = property on="Accept & Save" class="Bool (strict)"("DisabledEnum"=T19."Enabled" ("Disabled")) -> ()  [unwired: 2 in, 2 out]
        n756 = property on="Tab Control 5" class="TabCtl (strict)"("Value"=enum32{"OK", "NG"}."OK" ("Tab Control 5")) -> ()  [unwired: 2 in, 2 out]
      }
    }
    n757 = local read "Quit"() -> (w712:bool)
  }
  n758 = while {
    shift-right: [w780] -> _
    shift-left: "Enum - Selector" -> [w781]
    stop <- w782 stop-if-true
    # "Auto Start Logic Loop"
    n759 = case shown="\"Humidity & Temperature On\"" w781 {
      tunnel: [w785 w791 w818 w850 w880 Auto_Start_enum."Exit" ("Enum - Selector") Auto_Start_enum."Init" ("Enum - Selector")] -> w780
      frame "Init", Default {
        n760 = local read "Auto Start Test"() -> (w784:bool)
        n761 = Select(t=Auto_Start_enum."Humidity & Temperature On" ("Enum - Selector"), s=w784, f=Auto_Start_enum."Init") -> (s? t:f=w785:T15)
      }
      frame "Humidity & Temperature On" {
        n762 = stacked-sequence {
          tunnel: [_ _ _ _ _ _ Auto_Start_enum."Reach point" ("Enum - Selector")] -> w788
          frame #0 {
            w793 = T19."Disabled and Grayed Out" ("Disabled")
            w794 = TRUE ("Heater Button")
            n763 = property on="Humidity" class="Bool (strict)"("DisabledEnum"=w793) -> ()  [unwired: 2 in, 2 out]
            n764 = property on="Heater Button" class="Bool (strict)"("DisabledEnum"=w793) -> ()  [unwired: 2 in, 2 out]
            n765 = local write "Heater Button"(w794) -> ()
            n766 = local write "Humidity"(w794) -> ()
            n767 = property on="Heater Button" class="Bool (strict)"("Val(Sgnl)"=TRUE ("Value (Signaling)")) -> ()  [unwired: 2 in, 2 out]
          }
          frame #1 {
            n768 = Wait (ms)(milliseconds to wait=u32 3000) -> ()  [unwired: 1 out]
          }
          frame #2 {
            n769 = local read "Set Temp"() -> (w800:dbl)
            n770 = Number To Fractional String(number=w800, precision (6)=i16 2) -> (F-format string=w797:string)  [unwired: 2 in]
            n771 = Concatenate Strings("ST;" ("Command"), w797) -> (w798:string)
            n772 = local write "Due Write"(w798) -> ()
          }
          frame #3 {
            n773 = Wait (ms)(milliseconds to wait=u32 1500) -> ()  [unwired: 1 out]
          }
          frame #4 {
            (unwired) i16 2 ("precision (6)")
            n774 = local read "Write UNO"() -> (w802:string[])
            n775 = local read "Set Rh"() -> (w805:dbl)
            n776 = Number To Fractional String(number=w805) -> (F-format string=w806:string)  [unwired: 3 in]
            n777 = Concatenate Strings("M;" ("new element/subarray"), w806) -> (w807:string)
            n778 = local write "Due Write"("HE;1" ("Command")) -> ()
            n779 = Insert Into Array(array=w802, new element=w807) -> (w803:string[])  [unwired: 1 in]
            n780 = local write "Write UNO"(w803) -> ()
          }
          frame #5 {
            n781 = Wait (ms)(milliseconds to wait=u32 1500) -> ()  [unwired: 1 out]
          }
          frame #6 {
            w810 = TRUE ("Reach point temp")
            n782 = local write "Reach point Humidity"(w810) -> ()
            n783 = local write "Reach point temp"(w810) -> ()
          }
        }
        n784 = local read "Auto Start Test"() -> (w790:bool)
        n785 = Not(x=w790) -> (.not. x?=w789:bool)
        n786 = Select(t=Auto_Start_enum."close", s=w789, f=w788) -> (s? t:f=w791:T15)
      }
      frame "Reach point" {
        w819 = TRUE ("PAUSE")
        w827 = 1.0 ("y")
        w830 = 1.0 ("y")
        n787 = local read "Set Temp"() -> (w812:dbl)
        n788 = local read "Set Humidity:"() -> (w826:dbl)
        n789 = local read "Humidity ( %RH )"() -> (w831:dbl)
        n790 = Add(x=w812, y=w830) -> (x+y=w829:dbl)
        n791 = Subtract(x=w812, y=w830) -> (x-y=w828:dbl)
        n792 = Add(x=w826, y=w827) -> (x+y=w825:dbl)
        n793 = Subtract(x=w826, y=w827) -> (x-y=w824:dbl)
        n794 = local read "TEMP"() -> (w832:dbl)
        n795 = In Range and Coerce(upper limit=w825, x=w831, lower limit=w824) -> (In Range?=w813:bool)  [unwired: 1 out]
        n796 = In Range and Coerce(upper limit=w829, x=w832, lower limit=w828) -> (In Range?=w814:bool)  [unwired: 1 out]
        n797 = case shown="True" w813 {
          frame False {
          }
          frame True {
            n798 = case shown="True" "Reach point Humidity" {
              selector: "Reach point Humidity" -> [_ w838]
              frame False {
              }
              frame True {
                n799 = local read "EVENT LOG"() -> (w835:string)
                n800 = Not(x=w838) -> (.not. x?=w837:bool)
                n801 = local write "Reach point Humidity"(w837) -> ()
                n802 = call "Event Log.vi"("Content"="Target Humidity reached", "EVENT LOG"=w835) -> ("EVENT LOG"=w836:string)  [unwired: 8 in, 1 out]
                n803 = local write "EVENT LOG"(w836) -> ()
              }
            }
          }
        }
        n804 = case shown="True" w814 {
          frame False {
          }
          frame True {
            n805 = case shown="True" "Reach point temp" {
              selector: "Reach point temp" -> [_ w844]
              frame False {
              }
              frame True {
                n806 = local read "EVENT LOG"() -> (w841:string)
                n807 = Not(x=w844) -> (.not. x?=w843:bool)
                n808 = local write "Reach point temp"(w843) -> ()
                n809 = call "Event Log.vi"("Content"="Target Temperature reached", "EVENT LOG"=w841) -> ("EVENT LOG"=w842:string)  [unwired: 8 in, 1 out]
                n810 = local write "EVENT LOG"(w842) -> ()
              }
            }
          }
        }
        n811 = local read "Auto Start Test"() -> (w817:bool)
        n812 = And(x=w814, y=w813) -> (x .and. y?=w823:bool)
        n813 = Select(t=Auto_Start_enum."Maintain Stage" ("Enum - Selector"), s=w823, f=Auto_Start_enum."Reach point" ("Enum - Selector")) -> (s? t:f=w820:T15)
        n814 = Not(x=w817) -> (.not. x?=w816:bool)
        n815 = Select(t=Auto_Start_enum."close", s=w816, f=w820) -> (s? t:f=w818:T15)
        n816 = call "ELAPSED TIMER VI.vi"("RESET"=w819, "PAUSE"=w819) -> ()  [unwired: 7 in, 3 out]
      }
      frame "Maintain Stage" {
        w859 = 2.0 ("y")
        w858 = 1.0 ("y")
        # "Humidity and  temperatures Set Point  have been reached"
        n817 = local read "Set Temp"() -> (w845:dbl)
        n818 = local read "Set Humidity:"() -> (w862:dbl)
        n819 = local read "Humidity ( %RH )"() -> (w865:dbl)
        n820 = Add(x=w845, y=w858) -> (x+y=w864:dbl)
        n821 = Subtract(x=w845, y=w858) -> (x-y=w863:dbl)
        n822 = local read "TEMP"() -> (w866:dbl)
        n823 = Add(x=w862, y=w859) -> (x+y=w861:dbl)
        n824 = Subtract(x=w862, y=w859) -> (x-y=w860:dbl)
        n825 = In Range and Coerce(upper limit=w864, x=w866, lower limit=w863) -> (In Range?=w857:bool)  [unwired: 1 out]
        n826 = In Range and Coerce(upper limit=w861, x=w865, lower limit=w860) -> (In Range?=w856:bool)  [unwired: 1 out]
        n827 = And(x=w857, y=w856) -> (x .and. y?=w855:bool)
        n828 = Not(x=w855) -> (.not. x?=w854:bool)
        n829 = call "ELAPSED TIMER VI.vi"("TARGET"=60.0, "RESET"=w854, "PAUSE"=FALSE) -> ("ELAPSED INDICATION"=w851:bool)  [unwired: 6 in, 2 out]
        n830 = case shown="True" w851 {
          tunnel: w851 -> [_ w869]
          tunnel: [Auto_Start_enum."Maintain Stage" ("Enum - Selector") w868] -> w849
          frame False {
          }
          frame True {
            n831 = stacked-sequence {
              tunnel: w869 -> [_ _ _ _ _]
              tunnel: [_ _ _ _ Auto_Start_enum."Start Stage" ("Enum - Selector")] -> w868
              frame #0 {
                n832 = local read "EVENT LOG"() -> (w871:string)
                n833 = call "Event Log.vi"("Content"="Humidity and temperature set point has stabilized.", "EVENT LOG"=w871) -> ("EVENT LOG"=w872:string)  [unwired: 8 in, 1 out]
                n834 = local write "EVENT LOG"(w872) -> ()
              }
              frame #1 {
                n835 = Wait (ms)(milliseconds to wait=u32 100) -> ()  [unwired: 1 out]
              }
              frame #2 {
                n836 = local read "EVENT LOG"() -> (w875:string)
                n837 = call "Event Log.vi"("Content"="Auto Test Started", "EVENT LOG"=w875) -> ("EVENT LOG"=w876:string)  [unwired: 8 in, 1 out]
                n838 = local write "EVENT LOG"(w876) -> ()
              }
              frame #3 {
                w877 = TRUE ("RUN")
                n839 = local write "RUN"(w877) -> ()
                n840 = property on="Auto Start Temp" class="Bool (strict)"("Val(Sgnl)"=w877) -> ()  [unwired: 2 in, 2 out]
                "Auto Start Temp" <- w877
              }
              frame #4 {
              }
            }
          }
        }
        n841 = local read "Auto Start Test"() -> (w848:bool)
        n842 = Not(x=w848) -> (.not. x?=w847:bool)
        n843 = Select(t=Auto_Start_enum."close", s=w847, f=w849) -> (s? t:f=w850:T15)
      }
      frame "Start Stage" {
        w879 = TRUE ("PAUSE")
        n844 = local read "Auto Start Test"() -> (w884:bool)
        n845 = Not(x=w884) -> (.not. x?=w883:bool)
        n846 = Select(t=Auto_Start_enum."close" ("Enum - Selector"), s=w883, f=Auto_Start_enum."Start Stage" ("Enum - Selector")) -> (s? t:f=w880:T15)
        n847 = call "ELAPSED TIMER VI.vi"("RESET"=w879, "PAUSE"=w879) -> ()  [unwired: 7 in, 3 out]
      }
      frame "close" {
        w886 = FALSE ("Heater Button")
        n848 = local write "RUN"(w886) -> ()
        n849 = local write "Heater Button"(w886) -> ()
        n850 = local write "Humidity"(w886) -> ()
        n851 = local write "Auto Start Test"(w886) -> ()
        n852 = property on="Heater Button" class="Bool (strict)"("Val(Sgnl)"=FALSE ("Value (Signaling)")) -> ()  [unwired: 2 in, 2 out]
      }
      frame "Exit" {
      }
    }
    n853 = Wait (ms)(milliseconds to wait=u32 100) -> ()  [unwired: 1 out]
    n854 = local read "Quit"() -> (w782:bool)
  }
  n855 = property on="Service Password Log" class="Str"("Visible"=w21) -> ()  [unwired: 2 in, 2 out]
  n856 = property on="Password 3" class="Clust (strict)"("Visible"=w21) -> ()  [unwired: 2 in, 2 out]
  n857 = while {
    stop <- w915 stop-if-true
    w898 = errorcluster {"status"=FALSE, "code"=0, "source"=""} ("error in (no error) 3")
    # "this loop is for manual report generation"
    n858 = local read "Confirm Measrurement"() -> (w897:bool)
    n859 = case shown="True" w897 {
      selector: w897 -> [_ w1005]
      tunnel: errorcluster {"status"=FALSE, "code"=0, "source"=""} ("error in (no error) 3") -> [_ w1006]
      tunnel: [_ w1004] -> _
      frame False {
      }
      frame True {
        n860 = stacked-sequence {
          tunnel: w1006 -> [_ w1039 _]
          tunnel: w1005 -> [_ _ w1146]
          tunnel: [_ w1027 _] -> w1004
          frame #0 {
            n861 = String To Path(string="C:\\LAB-IQ\\Image Calibrate v01.dcf") -> (path=w1009:path)
            n862 = Open/Create/Replace File ("Open File")(file path (use dialog)=w1009) -> (refnum out=w1010:refnum<file>)  [unwired: 5 in, 2 out]
            n863 = for {
              N: 4 -> [_]
              tunnel: w1010 -> [w1016]
              i -> [w1012]
              n864 = Read from Text File ("Read File")(file (use dialog)=w1016) -> (text=w1017:string)  [unwired: 3 in, 3 out]
              n865 = String Subset(string=w1017, offset (0)=6, length (rest)=10 ("length (rest)")) -> (substring=w1013:string)
              n866 = Fract/Exp String To Number(string=w1013) -> (number=w1011:dbl)  [unwired: 3 in, 1 out]
              n867 = case shown="3" w1012 {
                tunnel: w1011 -> [w1018 w1019 _ w1020 _]
                frame 0 {
                  n868 = local write "5x Gain"(w1018) -> ()
                }
                frame 1 {
                  n869 = local write "10x Gain"(w1019) -> ()
                }
                frame 2 {
                }
                frame 3 {
                  n870 = local write "100x gain"(w1020) -> ()
                }
                frame 4, Default {
                }
              }
            }
          }
          frame #1 {
            n871 = local read "TEST STANDARD"() -> (w1022:T3)
            n872 = case shown="\"ISO 12156\"" w1022 {
              tunnel: ["ASTM D6079" "ISO 12156"] -> w1021
              frame "ASTM D6079", Default {
              }
              frame "ISO 12156" {
              }
            }
            n873 = call "IMAGE ANALYSIS.vi"("Enum"=POST_ANALYSIS_ENUM."GET MEASUREMENTS", "error in"=w1039) -> ("error out"=w1046:errorcluster)  [unwired: 8 in, 1 out]
            n874 = local read "Magnification :"() -> (w1032:string)
            n875 = call "Stall Data Flow.vim"("value in"=w1046, "milliseconds to wait"=u32 1000) -> ("value out"=w1045:errorcluster)  [unwired: 1 out]
            n876 = local read "Test File List :"() -> (w1043:string)
            n877 = case shown="\"10x\"" w1032 {
              tunnel: [w1082 w1083] -> w1030
              frame "5x", Default {
                n878 = local read "5x Gain"() -> (w1082:dbl)
              }
              frame "10x" {
                # "5x"
                n879 = local read "10x Gain"() -> (w1083:dbl)
              }
            }
            n880 = call "IMAGE ANALYSIS.vi"("Enum"=POST_ANALYSIS_ENUM."READ", "error in"=w1045) -> ("error out"=w1042:errorcluster, "data out"=w1033:string)  [unwired: 8 in]
            n881 = Match Pattern(string=w1033, regular expression="\"type\": ") -> (after substring=w1037:string)  [unwired: 1 in, 3 out]
            n882 = call "IMAGE PATH CREATION PY.vi"("error in (no error)"=w1042, "File Name :"=w1043) -> ("error out"=w1041:errorcluster, "File Path"=w1029:path, "File Path String:"=w1024:string)  [unwired: 7 in]
            n883 = Match Pattern(string=w1037, regular expression=",") -> (before substring=w1023:string)  [unwired: 1 in, 3 out]
            n884 = local read "Calibration Tab"() -> (w1026:enum32{"Measrument", "Calibrate"})
            n885 = call "Stall Data Flow.vim"("value in"=w1041, "milliseconds to wait"=u32 250) -> ("value out"=w1025:errorcluster)  [unwired: 1 out]
            n886 = Equal?(x=w1023, y="\"rectangle\"") -> (x = y?=w1034:bool)
            n887 = case shown="False" w1034 {
              tunnel: w1033 -> [w1088 w1143]
              tunnel: w1030 -> [_ w1134]
              tunnel: cluster{"major":dbl, "minor":dbl, "average":dbl} {"major"=0.0, "minor"=0.0, "average"=0.0} -> [w1086 w1130]
              tunnel: [w1085 w1127] -> w1028
              tunnel: w1023 -> [w1087 _]
              tunnel: w1030 -> [w1084 _]
              frame False {
                n888 = Equal?(x=w1087, y="\"line\"") -> (x = y?=w1089:bool)
                n889 = case shown="True" w1089 {
                  tunnel: w1088 -> [_ w1104]
                  tunnel: w1086 -> [w1091 w1103]
                  tunnel: [w1091 w1101] -> w1085
                  tunnel: w1084 -> [_ w1100]
                  frame False {
                  }
                  frame True {
                    w1099 = 0.0 ("Major Axis")
                    n890 = Match Pattern(string=w1104, regular expression="\"length_px\":") -> (after substring=w1102:string)  [unwired: 1 in, 3 out]
                    n891 = property on="Major Axis" class="DigNum (strict)"("Caption.Text"="") -> ()  [unwired: 2 in, 2 out]
                    n892 = property on="Minor Axis" class="DigNum (strict)"("Caption.Text"="") -> ()  [unwired: 2 in, 2 out]
                    n893 = property on="Average" class="DigNum (strict)"("Caption.Text"="Line") -> ()  [unwired: 2 in, 2 out]
                    n894 = Fract/Exp String To Number(string=w1102, default (0 dbl)=0.0 ("default (0 DBL)")) -> (number=w1098:dbl)  [unwired: 2 in, 1 out]
                    "Pixel Value" <- w1098
                    n895 = Multiply(x=w1098, y=w1100) -> (x*y=w1111:dbl)
                    n896 = Multiply(x=w1111, y=1000.0) -> (x*y=w1094:dbl)
                    n897 = Divide(x=w1094, y=1000.0) -> (x/y=w1097:dbl)
                    n898 = local write "Measurment (mm)"(w1097) -> ()
                    n899 = Bundle By Name(cluster=w1103, "average"=w1094) -> (w1101:cluster{"major":dbl, "minor":dbl, "average":dbl})
                    n900 = Number To Fractional String(number=w1094, precision (6)=i16 1) -> (F-format string=w1093:string)  [unwired: 2 in]
                    n901 = local write "Minor Axis"(w1099) -> ()
                    n902 = local write "Major Axis"(w1099) -> ()
                    n903 = Fract/Exp String To Number(string=w1093) -> (number=w1092:dbl)  [unwired: 3 in, 1 out]
                    n904 = local write "Average"(w1092) -> ()
                  }
                }
              }
              frame True {
                w1131 = 1000.0 ("y")
                w1137 = 0.0 ("default (0 DBL)")
                n905 = Match Pattern(string=w1143, regular expression=" \"width_px\":") -> (after substring=w1141:string)  [unwired: 1 in, 3 out]
